vi "EtherCAT Data Updated.vi"(8 "error in":errorcluster, 9 "Process Data Output":u8[](array[numeric]), 10 "Process Data Input":u8[](array[numeric])) -> (0 "error out":errorcluster)   [LabVIEW 2024, in "Hardware Controller.lvlib"]
doc: "Passes on the data received from the ethercat module after converting it.\n_____\nCreated using DQMH Event Scripter 7.0.0.1280."
uses:
  Hardware Controller.lvlib
  EtherCAT Data Updated Argument--cluster.ctl
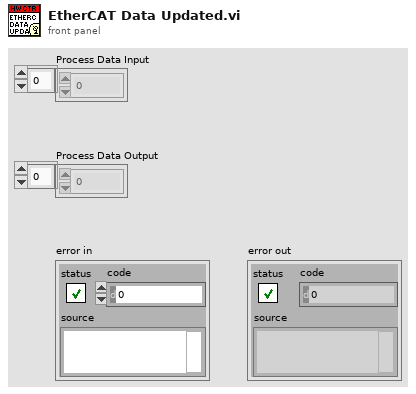
[diagram p1: front panel]
types:
  T1 = typedef "Hardware Controller.lvlib/EtherCAT Data Updated Argument--cluster.ctl" = cluster{"Process Data Input":u8[], "Process Data Output":u8[]}
  T2 = typedef "Hardware Controller.lvlib/Broadcast Events--cluster.ctl" = cluster{"Module Did Init":refnum<user-event>, "Status Updated":refnum<user-event>, "Error Reported":refnum<user-event>, "Module Did Stop":refnum<user-event>, "Update Module Execution Status":refnum<user-event>, "System State Updated":refnum<user-event>, "EtherCAT Data Updated":refnum<user-event>}
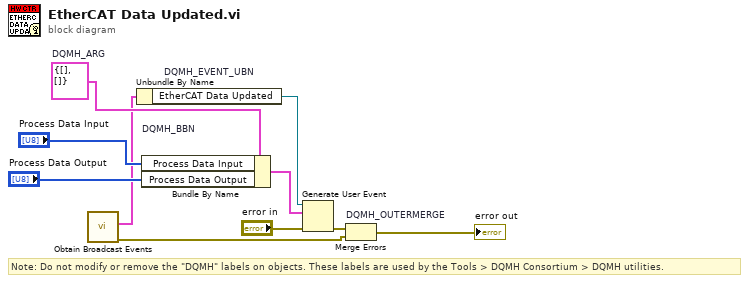
[diagram p0: block diagram]
diagram:
  w5 = T1 {"Process Data Input"=[], "Process Data Output"=[]}  # DQMH_ARG
  # "Note: Do not modify or remove the \"DQMH\" labels on objects. These labels are used by the Tools > DQMH Consortium > DQMH utilities."
  n1 = call "Obtain Broadcast Events.vi"() -> ("error out"=w2:errorcluster, "Hardware Controller Broadcast Events"=w1:T2)  [unwired: 10 in]
  n2 = Unbundle By Name "DQMH_EVENT_UBN"(w1) -> ("EtherCAT Data Updated"=w7:refnum<user-event>)
  n3 = Bundle By Name "DQMH_BBN"(cluster=w5, "Process Data Input"="Process Data Input", "Process Data Output"="Process Data Output") -> (w8:T1)
  n4 = Generate User Event(user event=w7, event data cluster=w8, error in="error in") -> (error out=w6:errorcluster)  [unwired: 1 in, 1 out]
  n5 = Merge Errors "DQMH_OUTERMERGE"(w6, w2) -> (→"error out":errorcluster)
